vi "Read Data Registers.vi"(11 "file (use dialog)":path) -> (0 "error out":errorcluster, 2 "Registers":u16[](array[numeric]), 3 "Config data":T2(array[cluster]))   [LabVIEW 2020, in "Sensor General Class.lvclass"]
uses:
  Sensor General Class.lvclass
panel:
  in  "Cluster 2":T1
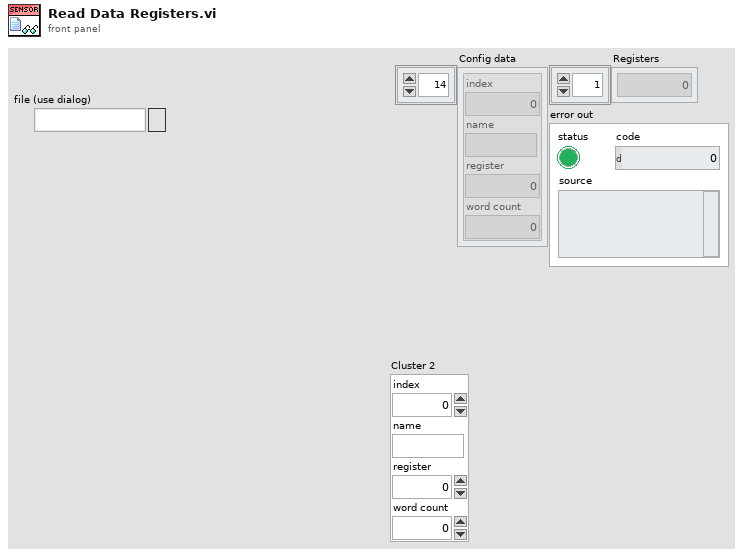
[diagram p1: front panel]
types:
  T1 = cluster{"index":i32, "name":string, "register":u16, "word count":u16}
  T2 = cluster{"index":i32, "name":string, "register":u16, "word count":u16}[]
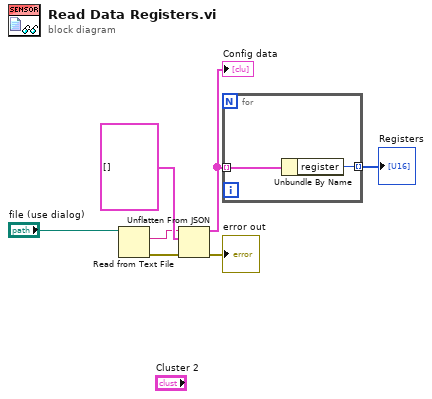
[diagram p0: block diagram]
diagram:
  n1 = Read from Text File(file (use dialog)="file (use dialog)") -> (text=w5:string, error out=w4:errorcluster)  [unwired: 3 in, 2 out]
  n2 = Unflatten From JSON(JSON string=w5, type and defaults=T2 [], error in (no error)=w4) -> (value=w3:T2, error out=→"error out":errorcluster)  [unwired: 4 in]
  "Config data" <- w3
  n3 = for {
    tunnel: w3 -> [w9] mode=indexing
    tunnel: [w8] -> w2 mode=indexing
    n4 = Unbundle By Name(w9) -> ("register"=w8:u16)
  }
  "Registers" <- w2
